vi "Semantic_Voice_Array_Msg.vi"(8 "error in (no error)":errorcluster caption="错误输入（无错误）", 10 "Semantic_Voice_Array":T1, 11 "ControlPanel输入":refnum<class "ControlPanel.lvclass">) -> (0 "error out":errorcluster caption="错误输出", 3 "ControlPanel输出":refnum<class "ControlPanel.lvclass">)   [LabVIEW 2014, in "ControlPanel.lvlib" / "ControlPanel.lvclass"]
uses:
  ControlPanel.lvclass
  ctl/Semantic_Voice_Array.ctl
  ControlPanel.lvclass/ControlPanel.ctl
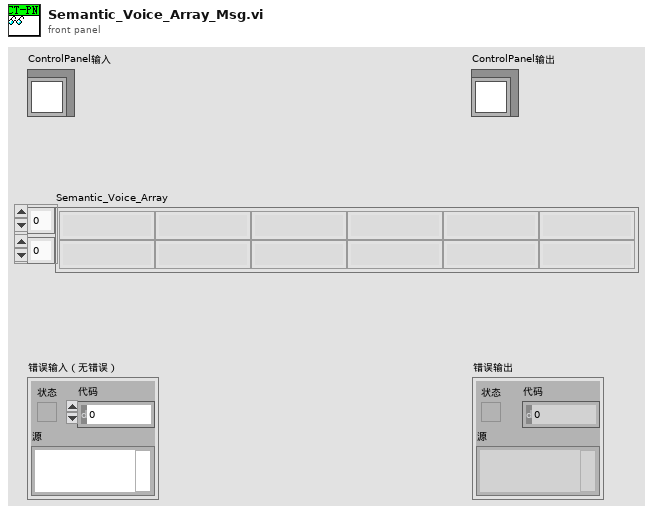
[diagram p1: front panel]
types:
  T1 = typedef "Semantic_Voice_Array.ctl" = string[][]
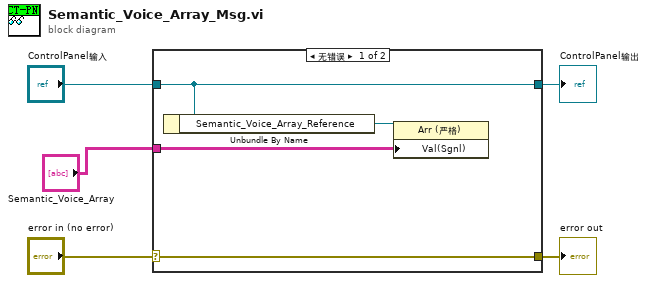
[diagram p0: block diagram]
diagram:
  n1 = case shown="无错误" "error in (no error)" {
    selector: "error in (no error)" -> [w9 w10]
    tunnel: [w9 w10] -> w4
    tunnel: [w8 w11] -> w2
    tunnel: "ControlPanel输入" -> [w8 w11]
    tunnel: "Semantic_Voice_Array" -> [w6 _]
    frame No Error {
      n2 = Unbundle By Name(w8) -> ("Semantic_Voice_Array_Reference"=w7:refnum<vi>)
      n3 = property class="Arr (严格)"(reference=w7, "Val(Sgnl)"=w6) -> ()  [unwired: 1 in, 2 out]
    }
    frame Error {
    }
  }
  "error out" <- w4
  "ControlPanel输出" <- w2
